vi "Windows UI C.vi"() -> ()   [LabVIEW 2015]
doc: "This is the primary host VI which reads and displays current value data from shared variables running on the target."
panel:
  out "Stage 3":bool
  out "Stage 2":bool
  out "Stage 1":bool
  in  "Stop UI":bool
  out "Amplitude":dbl format="%#_3g"
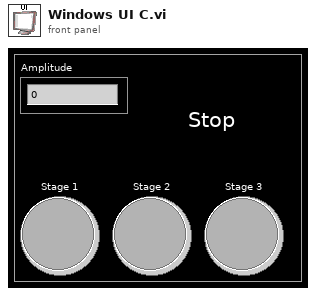
[diagram p1: front panel]
types:
  T1 = enum16{"big-endian, network order", "native, host order", "little-endian"}
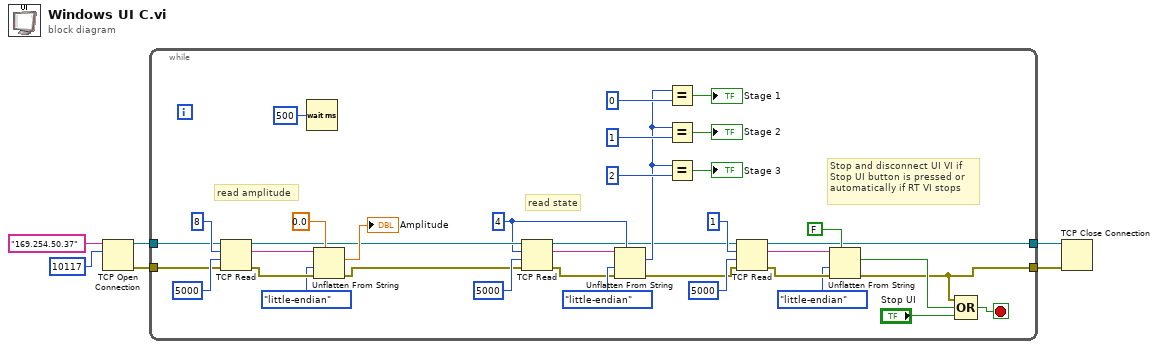
[diagram p0: block diagram]
diagram:
  n1 = TCP Open Connection(address="169.254.50.37", remote port or service name=u16 10117) -> (connection ID=w5:refnum<k5>, error out=w6:errorcluster)  [unwired: 3 in]
  n2 = while {
    tunnel: w6 -> [w30]
    tunnel: w5 -> [w31]
    tunnel: [w7] -> w2
    tunnel: [w8] -> w1
    stop <- w11 stop-if-true
    w21 = 4 ("bytes to read")
    # "read state"
    # "read amplitude"
    # "Stop and disconnect UI VI if \nStop UI button is pressed or \nautomatically if RT VI stops"
    n3 = TCP Read(connection ID=w31, bytes to read=8, error in (no error)=w30, 9:5000 ("timeout ms (25000)")) -> (connection ID out=w23:refnum<k5>, data out=w34:string, error out=w35:errorcluster)  [unwired: 1 in]
    n4 = Wait (ms)(milliseconds to wait=u32 500) -> ()  [unwired: 1 out]
    n5 = Unflatten From String(type=0.0, binary string=w34, byte order (0:big-endian, network order)=T1."little-endian", error in (no error)=w35) -> (value=→"Amplitude":dbl, error out=w22:errorcluster)  [unwired: 1 in, 1 out]
    n6 = TCP Read(connection ID=w23, bytes to read=w21, error in (no error)=w22, 9:5000 ("timeout ms (25000)")) -> (connection ID out=w14:refnum<k5>, data out=w26:string, error out=w25:errorcluster)  [unwired: 1 in]
    n7 = Unflatten From String(type=w21, binary string=w26, byte order (0:big-endian, network order)=T1."little-endian", error in (no error)=w25) -> (value=w20:i32, error out=w13:errorcluster)  [unwired: 1 in, 1 out]
    n8 = Equal?(x=w20, y=0 ("offset (0)")) -> (x = y?=→"Stage 1":bool)
    n9 = Equal?(x=w20, y=1 ("offset (0)")) -> (x = y?=→"Stage 2":bool)
    n10 = Equal?(x=w20, y=2 ("offset (0)")) -> (x = y?=→"Stage 3":bool)
    n11 = TCP Read(connection ID=w14, bytes to read=1, error in (no error)=w13, 9:5000 ("timeout ms (25000)")) -> (connection ID out=w8:refnum<k5>, data out=w16:string, error out=w17:errorcluster)  [unwired: 1 in]
    n12 = Unflatten From String(type=FALSE, binary string=w16, byte order (0:big-endian, network order)=T1."little-endian", error in (no error)=w17) -> (value=w9:bool, error out=w7:errorcluster)  [unwired: 1 in, 1 out]
    n13 = Compound Arithmetic op=OR(w7, w9, "Stop UI") -> (w11:bool)
  }
  n14 = TCP Close Connection(connection ID=w1, error in (no error)=w2) -> ()  [unwired: 1 in, 2 out]
